vi "update2dViewer.vi"(8 "error in (no error)":errorcluster, 9 "cam":u16, 10 "cur_nob":u32) -> (0 "error out":errorcluster)   [LabVIEW 2015, in "ESLSCDLL.lvlib"]
uses:
  ESLSCDLL.lvlib
  Globals.vi
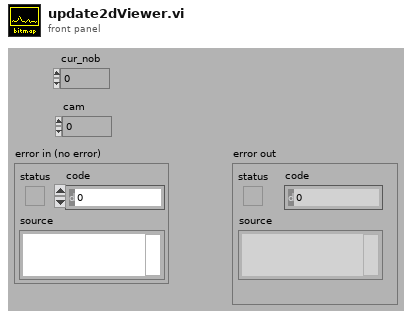
[diagram p1: front panel]
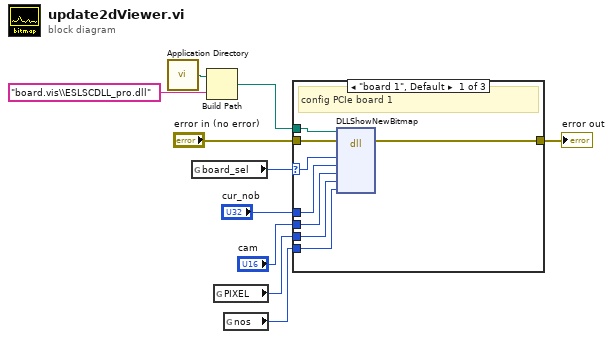
[diagram p0: block diagram]
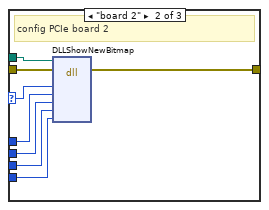
[diagram p2: hidden frame]
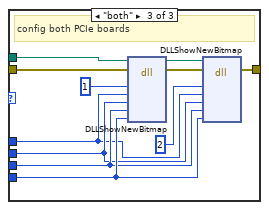
[diagram p3: hidden frame]
diagram:
  n1 = call <vilib>:"Application Directory.vi"() -> ("Application Directory"=w3:path)
  n2 = global read "Globals.vi" "board_sel"() -> (w5:enum32{"0", "board 1", "board 2", "both"})
  n3 = Build Path(base path=w3, name or relative path="board.vis\\ESLSCDLL_pro.dll") -> (appended path=w1:path)
  n4 = global read "Globals.vi" "PIXEL"() -> (w6:u32)
  n5 = global read "Globals.vi" "nos"() -> (w4:u32)
  n6 = case shown="\"board 1\", Default" w5 {
    selector: w5 -> [w18 w26 _]
    tunnel: "cur_nob" -> [w17 w25 w32]
    tunnel: "cam" -> [w16 w24 w33]
    tunnel: w6 -> [w15 w23 w34]
    tunnel: w4 -> [w14 w22 w35]
    tunnel: "error in (no error)" -> [w13 w21 w31]
    tunnel: [w12 w20 w29] -> w7
    tunnel: w1 -> [w11 w19 w28]
    frame "board 1", Default {
      # "config PCIe board 1"
      n7 = dll-call lib="C:/ENTW/PCIE/LV64/board.vis/ESLSCDLL_pro.dll" fn="DLLShowNewBitmap" ("lwlscdll.dll:DLLWriteLongS0")(path in=w11, error in=w13, "drvno"=w18, "cur_nob"=w17, "cam"=w16, "pixel"=w15, "nos"=w14) -> (error out=w12:errorcluster)  [unwired: 7 in, 1 out]
    }
    frame "board 2" {
      # "config PCIe board 2"
      n8 = dll-call lib="C:/ENTW/PCIE/LV64/board.vis/ESLSCDLL_pro.dll" fn="DLLShowNewBitmap" ("lwlscdll.dll:DLLWriteLongS0")(path in=w19, error in=w21, "drvno"=w26, "cur_nob"=w25, "cam"=w24, "pixel"=w23, "nos"=w22) -> (error out=w20:errorcluster)  [unwired: 7 in, 1 out]
    }
    frame "both" {
      # "config both PCIe boards"
      n9 = dll-call lib="C:/ENTW/PCIE/LV64/board.vis/ESLSCDLL_pro.dll" fn="DLLShowNewBitmap" ("lwlscdll.dll:DLLWriteLongS0")(path in=w28, error in=w31, "drvno"=u32 1, "cur_nob"=w32, "cam"=w33, "pixel"=w34, "nos"=w35) -> (path out=w27:path, error out=w30:errorcluster)  [unwired: 7 in]
      n10 = dll-call lib="C:/ENTW/PCIE/LV64/board.vis/ESLSCDLL_pro.dll" fn="DLLShowNewBitmap" ("lwlscdll.dll:DLLWriteLongS0")(path in=w27, error in=w30, "drvno"=u32 2, "cur_nob"=w32, "cam"=w33, "pixel"=w34, "nos"=w35) -> (error out=w29:errorcluster)  [unwired: 7 in, 1 out]
    }
  }
  "error out" <- w7
